vi "Get Class Topic Enqueuer.vi"(5 "Channel Class":refnum<class "Pub Sub Message Channel.lvclass">, 7 "Create if not exist? (T)":bool=TRUE, 8 "error in (no error)":errorcluster, 11 "Topic":refnum<class>) -> (0 "error out":errorcluster, 1 "Topic Enqueuer":refnum<class "Message Enqueuer.lvclass">, 2 "topic not found?":bool, 3 "Channel Out":refnum<class "Pub Sub Message Channel.lvclass">)   [LabVIEW 2020, in "Actor Pub Sub Channels.lvlib"]
uses:
  Actor Pub Sub Channels.lvlib
  <vilib>/ActorFramework/Message Enqueuer/Message Enqueuer.lvclass
  Pub Sub Message Channel/Pub Sub Message Channel.lvclass
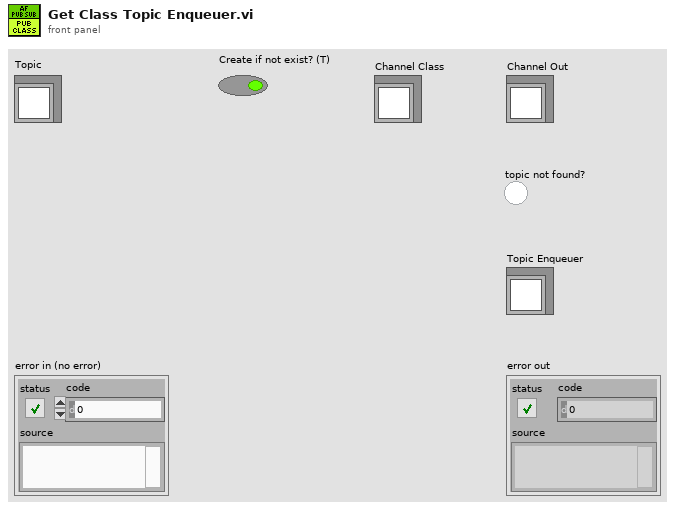
[diagram p1: front panel]
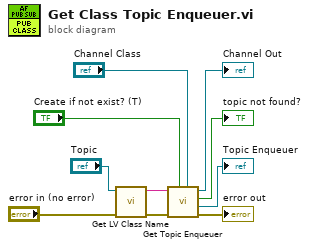
[diagram p0: block diagram]
diagram:
  n1 = call <vilib>:"Get LV Class Name.vi"("error in (no error)"="error in (no error)", "object"="Topic") -> ("error out"=w7:errorcluster, "class name"=w8:string)  [unwired: 8 in]
  n2 = call "Get Topic Enqueuer.vi"("Channel Class"="Channel Class", "Create if not exist? (T)"="Create if not exist? (T)", "error in (no error)"=w7, "Topic"=w8) -> ("error out"=→"error out":errorcluster, "Topic Enqueuer"=→"Topic Enqueuer":refnum<class "Message Enqueuer.lvclass">, "topic not found?"=→"topic not found?":bool, "Channel Out"=→"Channel Out":refnum<class "Pub Sub Message Channel.lvclass">)  [unwired: 4 in]
